vi "Write_xively_Wh.vi"(5 "thinfilm2":dbl, 6 "Thinfilm1":dbl, 7 "Poly Si 2":dbl, 8 "Poly Si 1":dbl, 9 "DSSC3":dbl, 10 "DSSC2":dbl, 11 "DSSC1":dbl) -> ()   [LabVIEW 2012]
uses:
  <vilib>/httpClient/LabVIEWHTTPClient.lvlib
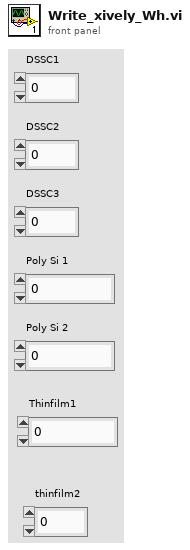
[diagram p1: front panel]
types:
  T1 = typedef "LabVIEWHTTPClient.lvlib/ClientHandle.ctl" = refnum<k1>
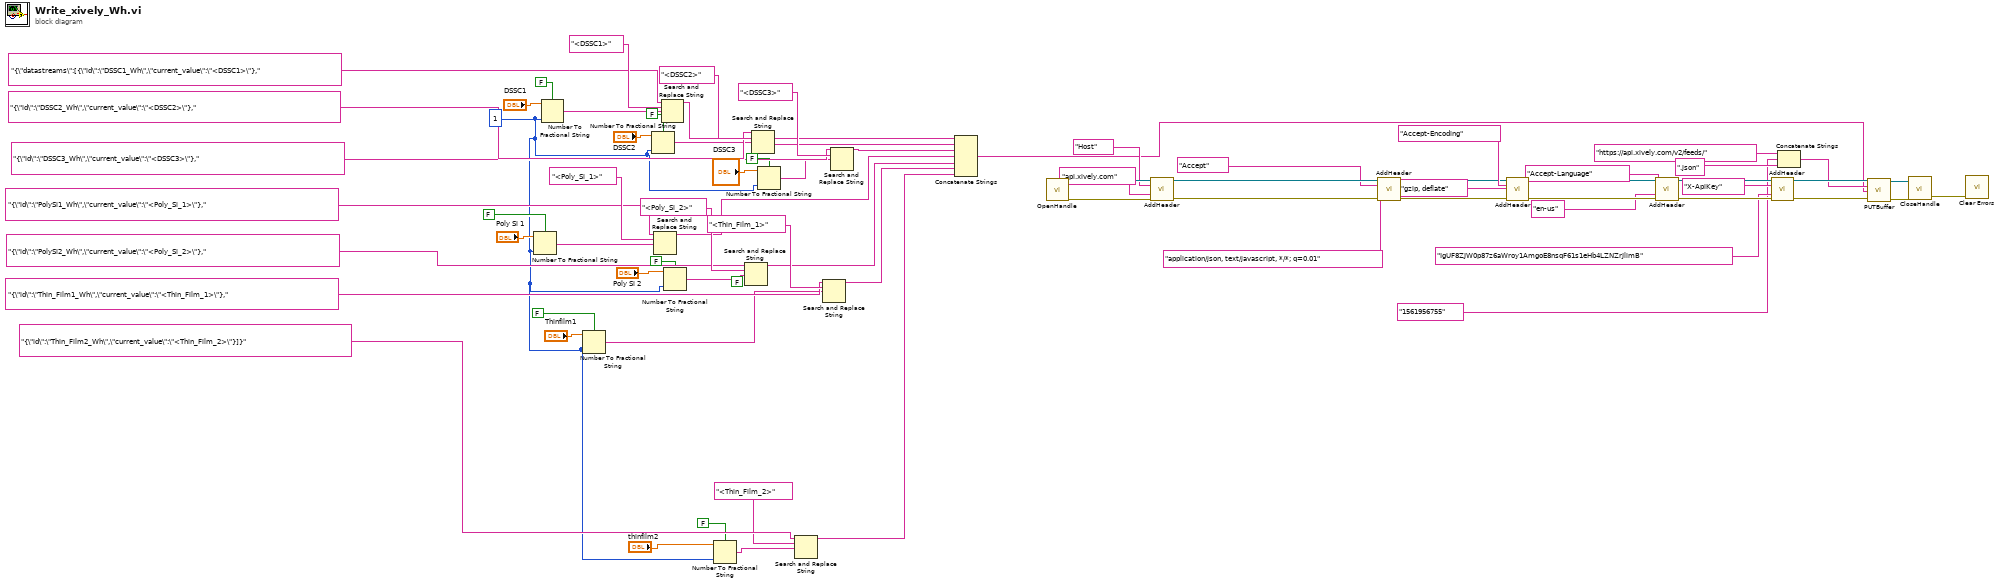
[diagram p0: block diagram]
diagram:
  (unwired) FALSE ("use system decimal point (T)")
  w2 = i16 1 ("precision (6)")
  n1 = Number To Fractional String(use system decimal point (T)=FALSE, number="Poly Si 1", precision (6)=w2) -> (F-format string=w35:string)  [unwired: 1 in]
  n2 = Number To Fractional String(use system decimal point (T)=FALSE, number="DSSC1", precision (6)=w2) -> (F-format string=w50:string)  [unwired: 1 in]
  n3 = Number To Fractional String(use system decimal point (T)=FALSE, number="Thinfilm1", precision (6)=w2) -> (F-format string=w3:string)  [unwired: 1 in]
  n4 = Number To Fractional String(use system decimal point (T)=FALSE, number="DSSC2", precision (6)=w2) -> (F-format string=w28:string)  [unwired: 1 in]
  n5 = Search and Replace String(input string="{\"id\":\"PolySi1_Wh\",\"current_value\":\"<Poly_Si_1>\"},", search string="<Poly_Si_1>", replace string=w35) -> (result string=w24:string)  [unwired: 5 in, 3 out]
  n6 = Search and Replace String(input string="{\"datastreams\":[{\"id\":\"DSSC1_Wh\",\"current_value\":\"<DSSC1>\"},", search string="<DSSC1>", replace string=w50) -> (result string=w16:string)  [unwired: 5 in, 3 out]
  n7 = Number To Fractional String(use system decimal point (T)=FALSE, number="Poly Si 2", precision (6)=w2) -> (F-format string=w21:string)  [unwired: 1 in]
  n8 = Number To Fractional String(use system decimal point (T)=FALSE, number="thinfilm2", precision (6)=w2) -> (F-format string=w18:string)  [unwired: 1 in]
  n9 = Search and Replace String(input string="{\"id\":\"PolySi2_Wh\",\"current_value\":\"<Poly_Si_2>\"},", search string="<Poly_Si_2>", replace string=w21) -> (result string=w23:string)  [unwired: 5 in, 3 out]
  n10 = Search and Replace String(input string="{\"id\":\"DSSC2_Wh\",\"current_value\":\"<DSSC2>\"},", search string="<DSSC2>", replace string=w28) -> (result string=w38:string)  [unwired: 5 in, 3 out]
  n11 = Number To Fractional String(use system decimal point (T)=FALSE, number="DSSC3", precision (6)=w2) -> (F-format string=w27:string)  [unwired: 1 in]
  n12 = Search and Replace String(input string="{\"id\":\"Thin_Film2_Wh\",\"current_value\":\"<Thin_Film_2>\"}]}", search string="<Thin_Film_2>", replace string=w18) -> (result string=w8:string)  [unwired: 5 in, 3 out]
  n13 = Search and Replace String(input string="{\"id\":\"Thin_Film1_Wh\",\"current_value\":\"<Thin_Film_1>\"},", search string="<Thin_Film_1>", replace string=w3) -> (result string=w22:string)  [unwired: 5 in, 3 out]
  n14 = Search and Replace String(input string="{\"id\":\"DSSC3_Wh\",\"current_value\":\"<DSSC3>\"},", search string="<DSSC3>", replace string=w27) -> (result string=w37:string)  [unwired: 5 in, 3 out]
  n15 = Concatenate Strings(w16, w38, w37, w24, w23, w22, w8) -> (w15:string)
  n16 = call <vilib>:"OpenHandle.vi"() -> ("client handle out"=w69:T1, "error out"=w68:errorcluster)  [unwired: 14 in]
  n17 = call <vilib>:"AddHeader.vi"("client handle"=w69, "header"="Host", "value"="api.xively.com", "error in (no error)"=w68) -> ("client handle out"=w65:T1, "error out"=w64:errorcluster)  [unwired: 10 in]
  n18 = call <vilib>:"AddHeader.vi"("client handle"=w65, "header"="Accept", "value"="application/json, text/javascript, */*; q=0.01", "error in (no error)"=w64) -> ("client handle out"=w60:T1, "error out"=w59:errorcluster)  [unwired: 10 in]
  n19 = call <vilib>:"AddHeader.vi"("client handle"=w60, "header"="Accept-Encoding", "value"="gzip, deflate", "error in (no error)"=w59) -> ("client handle out"=w57:T1, "error out"=w56:errorcluster)  [unwired: 10 in]
  n20 = call <vilib>:"AddHeader.vi"("client handle"=w57, "header"="Accept-Language", "value"="en-us", "error in (no error)"=w56) -> ("client handle out"=w53:T1, "error out"=w52:errorcluster)  [unwired: 10 in]
  n21 = call <vilib>:"AddHeader.vi"("client handle"=w53, "header"="X-ApiKey", "value"="IgUF8ZJW0p87z6aWroy1AmgoE8nsqF61s1eHb4LZNZrJlimB" ("API Key"), "error in (no error)"=w52) -> ("client handle out"=w72:T1, "error out"=w71:errorcluster)  [unwired: 10 in]
  n22 = Concatenate Strings("https://api.xively.com/v2/feeds/" ("url"), "1561956755" ("Feed ID"), ".json" ("string")) -> (w47:string)
  n23 = call <vilib>:"PUTBuffer.vi"("client handle"=w72, "url"=w47, "buffer"=w15, "error in (no error)"=w71) -> ("client handle out"=w46:T1, "error out"=w45:errorcluster)  [unwired: 8 in, 2 out]
  n24 = call <vilib>:"CloseHandle.vi"("client handle"=w46, "error in (no error)"=w45) -> ("error out"=w14:errorcluster)  [unwired: 13 in]
  n25 = call <vilib>:"Clear Errors.vi"("error in (no error)"=w14) -> ()  [unwired: 6 in, 1 out]
